vi "Mini Configure Experiment.vi"(5 "Control Experiment in":refnum<class "Control Experiment.lvclass">, 6 "Username":string, 8 "error in (no error)":errorcluster, 9 "Device Description":string, 10 "Device Name":string, 11 "Base Path":path) -> (0 "error out":errorcluster, 3 "Control Experiment out":refnum<class "Control Experiment.lvclass">)   [LabVIEW 2019, in "Control Experiment.lvclass"]
uses:
  Control Experiment.lvclass
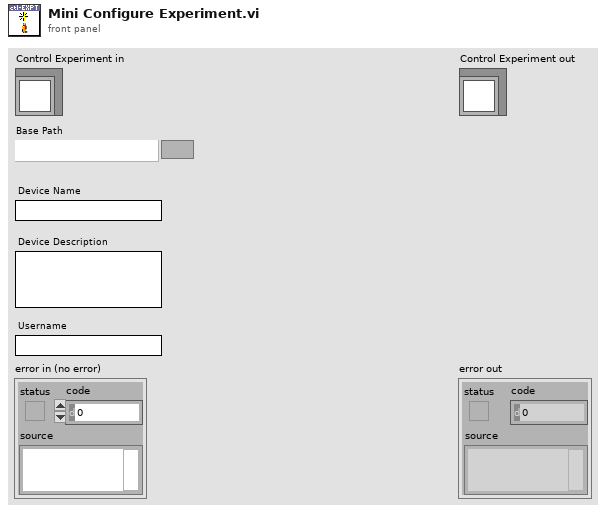
[diagram p1: front panel]
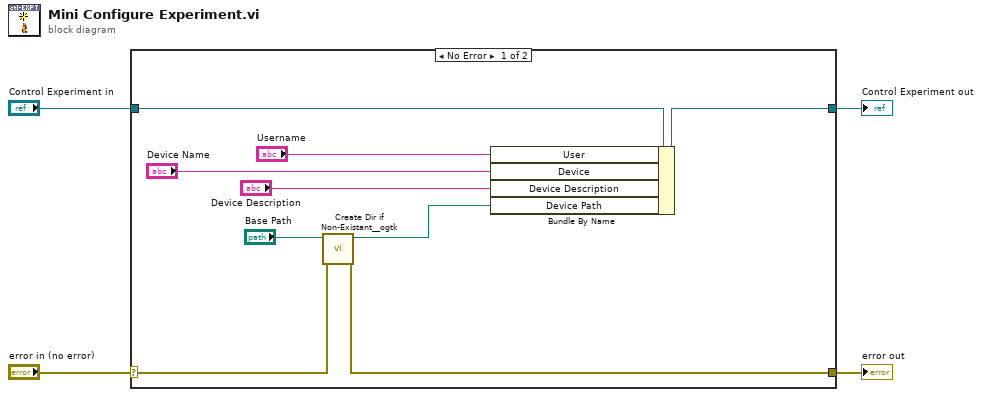
[diagram p0: block diagram]
diagram:
  n1 = case shown="No Error" "error in (no error)" {
    selector: "error in (no error)" -> [w7 w15]
    tunnel: [w6 w15] -> w3
    tunnel: [w13 w14] -> w1
    tunnel: "Control Experiment in" -> [w12 w14]
    frame No Error {
      n2 = call <userlib>:"Create Dir if Non-Existant__ogtk.vi"("error in (no error)"=w7, "Directory Path"="Base Path") -> ("error out"=w6:errorcluster, "dup Directory Path"=w8:path)  [unwired: 7 in, 1 out]
      n3 = Bundle By Name(cluster=w12, "User"="Username", "Device"="Device Name", "Device Description"="Device Description", "Device Path"=w8) -> (w13:refnum<class "Control Experiment.lvclass">)
    }
    frame Error {
    }
  }
  "error out" <- w3
  "Control Experiment out" <- w1
